vi "GetSelectedColumnRowIndex.vi"(0 "reference in":refnum<class "DataGridView.lvclass">, 11 "error in (no error)":errorcluster) -> (4 "reference out":refnum<class "DataGridView.lvclass">, 6 "ColumnIndex":i32, 8 "RowIndex":i32, 15 "error out":errorcluster)   [LabVIEW 2018, in "DataGridView.lvclass"]
doc: "Gets the index for the columns and the rows of the selected cell"
uses:
  DataGridView.lvclass
  System.Windows.Forms
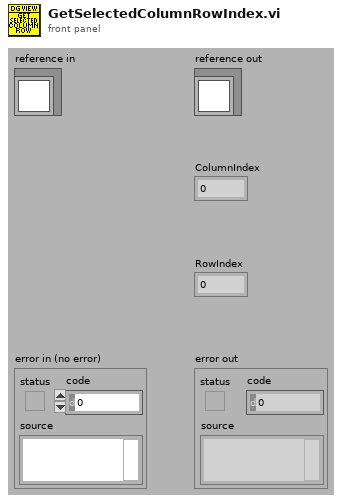
[diagram p1: front panel]
types:
  T1 = typedef "DataGridView.lvclass/ObjectAttributes.ctl" = cluster{"DataGridView":refnum<k24>, "SelectionChangedEvent":refnum<user-event>, "SelectionChanged callback ref":refnum<k27>, "LastSelectedRowIndex":i32}
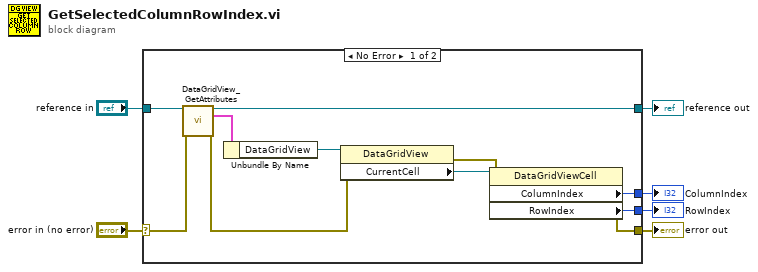
[diagram p0: block diagram]
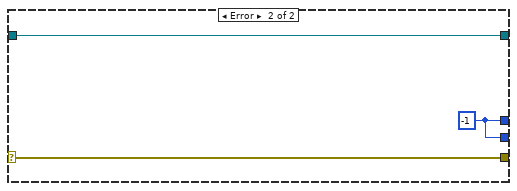
[diagram p2: hidden frame]
diagram:
  n1 = case shown="No Error" "error in (no error)" {
    selector: "error in (no error)" -> [w17 w20]
    tunnel: [w7 w20] -> w5
    tunnel: [w14 w19] -> w3
    tunnel: "reference in" -> [w15 w19]
    tunnel: [w10 w18] -> w2
    tunnel: [w9 w18] -> w1
    frame No Error {
      n2 = call "DataGridView_GetAttributes.vi"("reference in"=w15, "error in (no error)"=w17) -> ("reference out"=w14:refnum<class "DataGridView.lvclass">, "Data"=w16:T1, "error out"=w12:errorcluster)  [unwired: 10 in, 1 out]
      n3 = Unbundle By Name(w16) -> ("DataGridView"=w13:refnum<k24>)
      n4 = property class="DataGridView"(reference=w13, error in=w12) -> (error out=w8:errorcluster, "CurrentCell"=w11:refnum<k24>)  [unwired: 1 out]
      n5 = property class="DataGridViewCell"(reference=w11, error in=w8) -> (error out=w7:errorcluster, "ColumnIndex"=w10:i32, "RowIndex"=w9:i32)  [unwired: 1 out]
    }
    frame Error {
      w18 = -1 ("ColumnIndex")
    }
  }
  "error out" <- w5
  "reference out" <- w3
  "ColumnIndex" <- w2
  "RowIndex" <- w1
